vi "Load Grid Plot AER.vi"() -> ()   [LabVIEW 2013]
uses:
  AER/AER.lvclass
  Cerebellum/Cerebellum.lvclass
  <vilib>/Utility/miscctls.llb/LVBoundsTypeDef.ctl
  Cube/Grid.lvclass
  Controls/Type of Neuron.ctl
  Controls/Neuron Info.ctl
panel:
  out "error out":errorcluster
  out "PreIDs [i]":i32[](array[numeric])
  out "NoPre [i]":i32
  out "No N acc":i32[](array[numeric])
  in  "N":i32
  out "2D Picture":picture
  in  "stop":bool
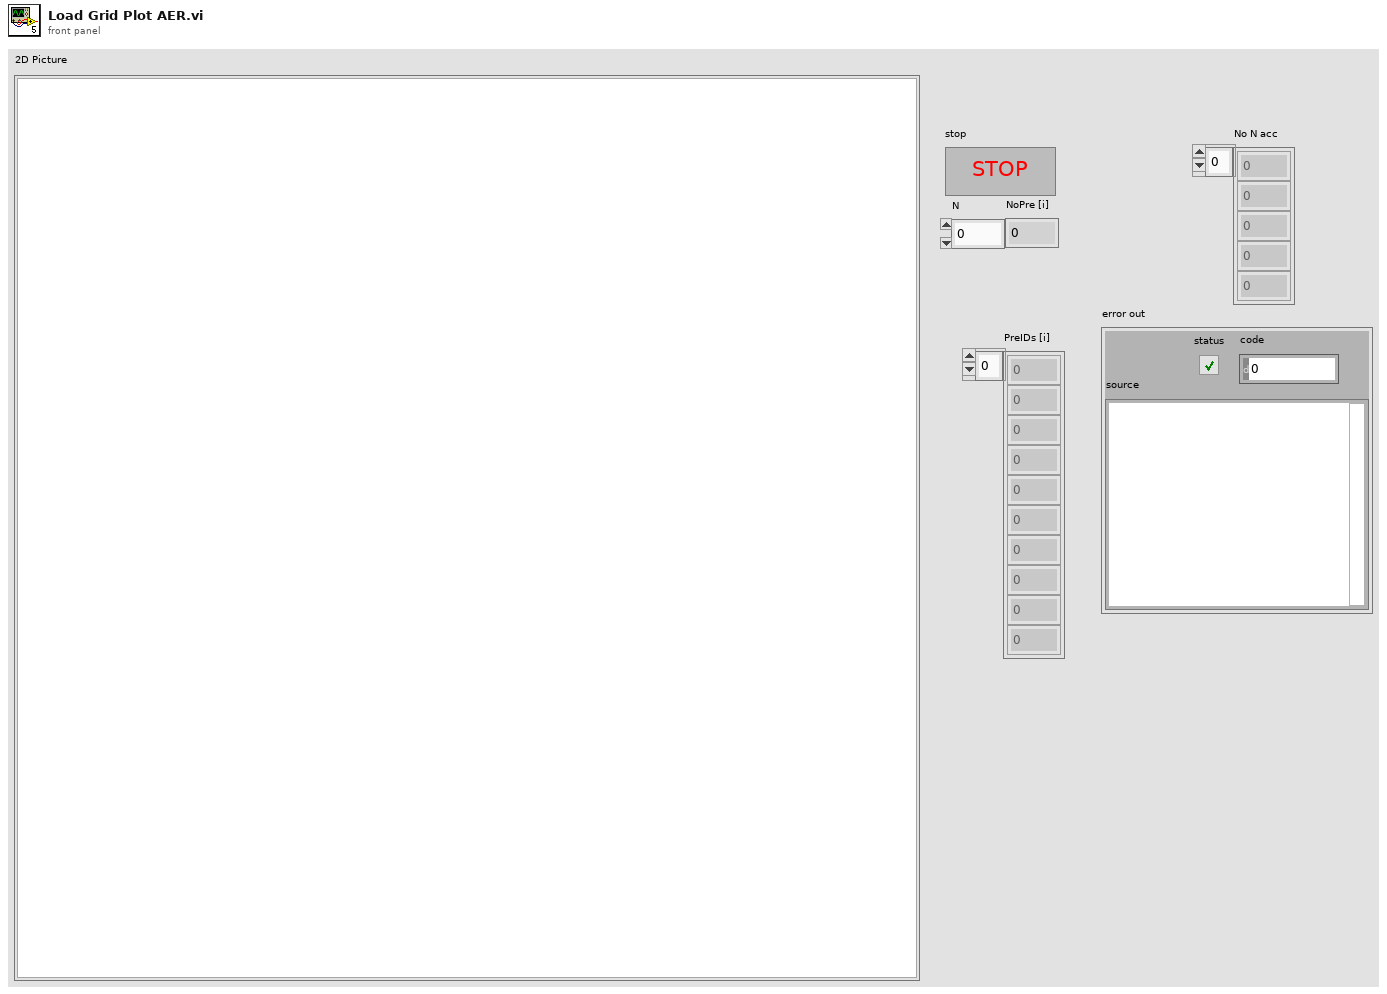
[diagram p1: front panel]
types:
  T1 = typedef "Neuron Info.ctl" = cluster{"N":i32, "Radius":dbl, "Type":T2, "Color":u32}[]
  T2 = typedef "Type of Neuron.ctl" = enum16{"MF", "BA", "GO", "GC", "PC", "LU", "Glia (Dummy)"}
  T3 = typedef "LVBoundsTypeDef.ctl" = cluster{"Width":u32, "Height":u32}
  T4 = cluster{"Width":u16, "Style":enum32{"Solid", "Dash", "Dot", "DashDot", "DashDotDot"}}
  T5 = enum32{"Solid", "Dash", "Dot", "DashDot", "DashDotDot"}
  T6 = cluster{dbl, "Style":enum32{"Solid", "Dash", "Dot", "DashDot", "DashDotDot"}}
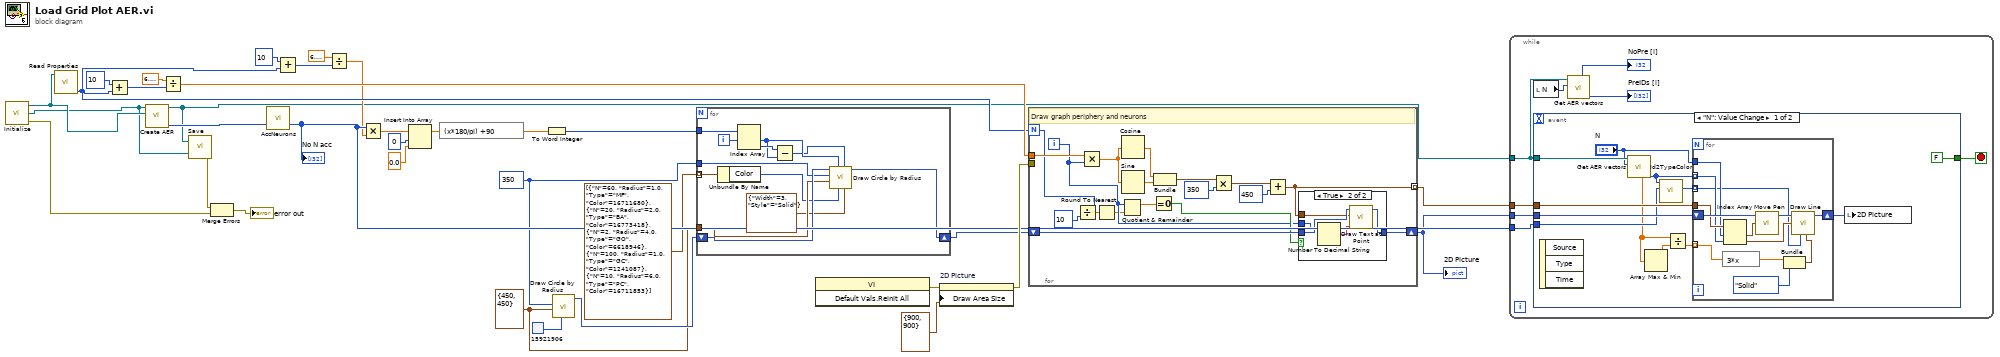
[diagram p0: block diagram]
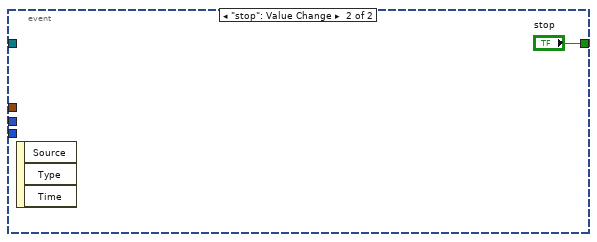
[diagram p2: hidden frame]
diagram:
  w16 = cluster{"horizontal":i16, "vertical":i16} {"horizontal"=450, "vertical"=450} ("pixel center")
  w15 = i16 350 ("radius")
  n1 = call "Initialize.vi"() -> ("Grid out"=w6:refnum<class "Grid.lvclass">, "Synapses out"=w2:refnum<class "Synapses.lvclass">, "error out"=w1:errorcluster)  [unwired: 1 in]
  n2 = call "Read Properties.vi"("Grid in"=w6) -> ("No Neurons"=w21:i32)  [unwired: 6 in, 4 out]
  n3 = Add(x=10, y=w21) -> (x+y=w27:i32)
  n4 = call "Create AER.vi"("Grid.lvclass"=w6, "Synapses in"=w2) -> ("No N"=w34:i32[], "AER.lvclass"=w4:refnum<class "AER.lvclass">)  [unwired: 6 in, 2 out]
  n5 = Divide(x=6.283185307179586, y=w27) -> (x/y=w31:dbl)
  n6 = call "Save.vi"("Synapses in"=w2, "AER in"=w4) -> ("error out"=w3:errorcluster)
  n7 = Merge Errors(w3, w1) -> (→"error out":errorcluster)
  n8 = call "AccNeurons.vi"("No N"=w34) -> ("No N acc"=w20:i32[])  [unwired: 2 in]
  "No N acc" <- w20
  n9 = Add(x=10, y=w21) -> (x+y=w22:i32)
  n10 = Divide(x=6.283185307179586, y=w22) -> (x/y=w19:dbl)
  n11 = Multiply(x=w20, y=w19) -> (x*y=w11:dbl[])
  n12 = Insert Into Array(array=w11, index=0, new element=0.0 ("new element/subarray")) -> (w10:dbl[])
  n13 = expression code="(x*180/pi) +90"(w10) -> (w9:dbl[])
  n14 = To Word Integer(number=w9) -> (16bit integer=w7:i16[])
  n15 = call <vilib>:"Draw Circle by Radius.vi"("color(black)"=u32 15921906, "pixel center"=w16, "radius"=w15) -> ("new picture"=w17:picture)  [unwired: 8 in]
  n16 = for {
    tunnel: w16 -> [w45]
    tunnel: w15 -> [w44]
    tunnel: w7 -> [w41]
    tunnel: T1 [{"N"=60, "Radius"=1.0, "Type"=enum."MF", "Color"=16711680}, {"N"=20, "Radius"=2.0, "Type"=enum."BA", "Color"=16773418}, {"N"=2, "Radius"=4.0, "Type"=enum."GO", "Color"=6618946}, {"N"=100, "Radius"=1.0, "Type"=enum."GC", "Color"=1241087}, {"N"=10, "Radius"=6.0, "Type"=enum."PC", "Color"=16711853}] ("Neurons Info") -> [w39] mode=indexing
    shift-right: [w43] -> w14
    shift-left: w17 -> [w46]
    i -> [w40]
    n17 = Unbundle By Name(w39) -> ("Color"=w38:u32)
    n18 = Index Array(array=w41, index #1=w40) -> (element #1=w36:i16, element #2=w37:i16)  [unwired: 1 in]
    n19 = Subtract(x=w37, y=w36) -> (x-y=w35:i16)
    n20 = call <vilib>:"Draw Circle by Radius.vi"("pen"=T4 {"Width"=3, "Style"=enum."Solid"}, "arc size(360)"=w35, "color(black)"=w38, "start angle(0)"=w36, "pixel center"=w45, "radius"=w44, "picture"=w46) -> ("new picture"=w43:picture)  [unwired: 4 in]
  }
  n21 = invoke class="VI" method="Default Vals.Reinit All"() -> (error out=w25:errorcluster)  [unwired: 3 in, 2 out]
  n22 = property on="2D Picture" class="Pict"(error in=w25, "Draw Area Size"=T3 {"Width"=900, "Height"=900}) -> (error out=w29:errorcluster)  [unwired: 1 in, 1 out]
  n23 = for {
    N: w21 -> [w51]
    shift-right: [w56] -> w18
    shift-left: w14 -> [w60]
    tunnel: w31 -> [w59]
    tunnel: [w57] -> w28 mode=indexing
    tunnel: w29 -> [_]
    i -> [w48]
    # "Draw graph periphery and neurons"
    n24 = Divide(x=w51, y=10 ("x")) -> (x/y=w50:dbl)
    n25 = Multiply(x=w59, y=w48) -> (x*y=w54:dbl)
    n26 = Round To Nearest(number=w50) -> (nearest integer value=w47:dbl)
    n27 = Quotient & Remainder(x=w48, y=w47) -> (x-y*floor(x/y)=w53:dbl)  [unwired: 1 out]
    n28 = Cosine(x=w54) -> (cos(x)=w55:dbl)
    n29 = Sine(x=w54) -> (sin(x)=w64:dbl)
    n30 = Equal To 0?(x=w53) -> (x = 0?=w52:bool)
    n31 = Bundle(w55, w64) -> (w58:cluster{dbl, dbl})  [unwired: 1 in]
    n32 = Multiply(x=w58, y=i16 350 ("vertical")) -> (x*y=w63:cluster{dbl, dbl})
    n33 = Add(x=w63, y=i16 450 ("vertical")) -> (x+y=w57:cluster{dbl, dbl})
    n34 = case shown="True" w52 {
      tunnel: w60 -> [w65 w70]
      tunnel: [w65 w69] -> w56
      tunnel: w48 -> [_ w68]
      tunnel: w57 -> [_ w66]
      frame False {
      }
      frame True {
        n35 = Number To Decimal String(number=w68) -> (decimal integer string=w67:string)  [unwired: 1 in]
        n36 = call <vilib>:"Draw Text at Point.vi"("text"=w67, "origin"=w66, "picture"=w70) -> ("new picture"=w69:picture)  [unwired: 7 in, 1 out]
      }
    }
  }
  "2D Picture" <- w18
  n37 = while {
    tunnel: w4 -> [w74]
    tunnel: w28 -> [w78]
    tunnel: w18 -> [w76]
    tunnel: w20 -> [w71]
    stop <- w77 stop-if-true
    n38 = local read "N"() -> (w72:i32)
    n39 = event shown="[0] \"N\": Value Change" {
      selector: _ -> [_ _]
      dyn-events: _ -> [_ _]
      timeout: _ -> [_ _]
      tunnel: w74 -> [w90 _]
      tunnel: w78 -> [w89 _]
      tunnel: w76 -> [w88 _]
      tunnel: [FALSE "stop"] -> w77
      tunnel: w71 -> [w83 _]
      event "N": Value Change {
        n40 = event-data() -> ()  [unwired: 1 in, 3 out]
        n41 = call "Get AER vectors.vi"("ID [i]"="N", "AER in"=w90) -> ("PreIDs [i]"=w84:i32[], "W[i]"=w81:dbl[])  [unwired: 4 in, 4 out]
        n42 = Array Max & Min(array=w81) -> (max value=w79:dbl)  [unwired: 3 out]
        n43 = call "Id2TypeColor.vi"("Acc N"=w83, "PreIds"=w84) -> ("Colors"=w82:u32[])  [unwired: 8 in, 1 out]
        n44 = Divide(x=w81, y=w79) -> (x/y=w80:dbl[])
        n45 = for {
          tunnel: w84 -> [w96] mode=indexing
          tunnel: w89 -> [w100]
          shift-right: [w101] -> w85
          shift-left: w88 -> [w103]
          tunnel: "N" -> [w99]
          tunnel: w82 -> [w95] mode=indexing
          tunnel: w80 -> [w93] mode=indexing
          n46 = expression code="3*x"(w93) -> (w92:dbl)
          n47 = Index Array(array=w100, index #1=w99, index #2=w96) -> (element #1=w98:cluster{dbl, dbl}, element #2=w97:cluster{dbl, dbl})
          n48 = call <vilib>:"Move Pen.vi"("new position"=w98, "picture"=w103) -> ("new picture"=w102:picture)  [unwired: 3 in]
          n49 = Bundle(w92, "Style"=T5."Solid") -> (w94:T6)  [unwired: 1 in]
          n50 = call <vilib>:"Draw Line.vi"("picture"=w102, "end point"=w97, "color(black)"=w95, "pen"=w94) -> ("new picture"=w101:picture)  [unwired: 5 in]
        }
        n51 = local write "2D Picture"(w85) -> ()
      }
      event "stop": Value Change {
        n52 = event-data() -> ()  [unwired: 1 in, 3 out]
      }
    }
    n53 = call "Get AER vectors.vi"("ID [i]"=w72, "AER in"=w74) -> ("PreIDs [i]"=→"PreIDs [i]":i32[], "NoPre [i]"=→"NoPre [i]":i32)  [unwired: 4 in, 4 out]
  }
